vi "Get Column Names.vi"(8 "error in (no error)":errorcluster, 11 "Table in":refnum<class "Table.lvclass">) -> (0 "error out":errorcluster, 1 "Key Names":string[](array[string]), 2 "Column Names":string[](array[string]), 3 "Table out":refnum<class "Table.lvclass">)   [LabVIEW 2020, in "Table.lvlib" / "Table.lvclass"]
uses:
  Table.lvclass
  Table.lvclass/Table.ctl
  Column Interface/Column Interface Class/Column Interface.lvclass
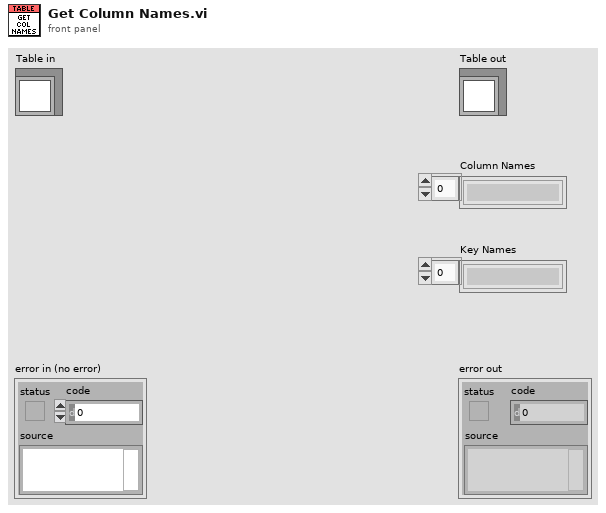
[diagram p1: front panel]
types:
  T1 = map{string, refnum<class "Column Interface.lvclass">}
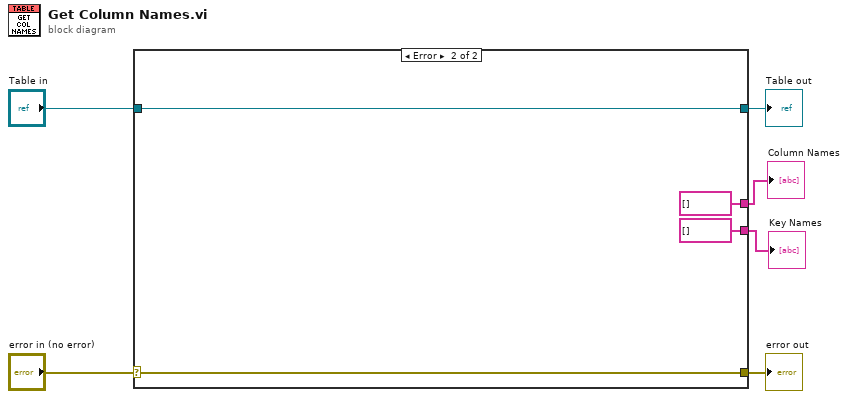
[diagram p0: block diagram]
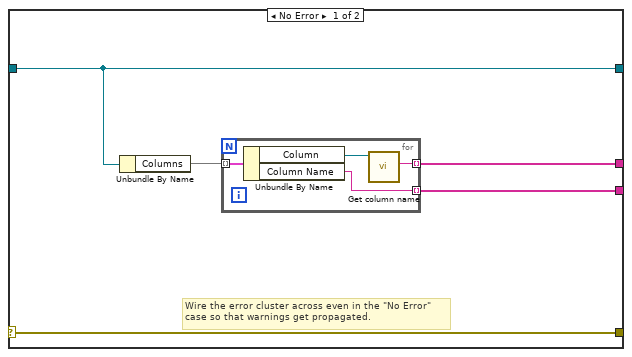
[diagram p2: hidden frame]
diagram:
  n1 = case shown="Error" "error in (no error)" {
    selector: "error in (no error)" -> [w11 w19]
    tunnel: [w11 w19] -> w5
    tunnel: [w10 w18] -> w3
    tunnel: "Table in" -> [w10 w18]
    tunnel: [w8 string[] []] -> w2
    tunnel: [w7 string[] []] -> w1
    frame No Error {
      # "Wire the error cluster across even in the \"No Error\"\ncase so that warnings get propagated."
      n2 = Unbundle By Name(w10) -> ("Columns"=w9:T1)
      n3 = for {
        tunnel: w9 -> [w15] mode=indexing
        tunnel: [w14] -> w7 mode=indexing
        tunnel: [w12] -> w8 mode=indexing
        n4 = Unbundle By Name(w15) -> ("Column"=w13:refnum<class "Column Interface.lvclass">, "Column Name"=w14:string)
        n5 = call-dynamic "Get column name.vi"("Column Interface in"=w13) -> ("Name"=w12:string)  [unwired: 8 in, 2 out]
      }
    }
    frame Error {
    }
  }
  "error out" <- w5
  "Table out" <- w3
  "Key Names" <- w1
  "Column Names" <- w2
